vi "Create Message Classes for Actor.vi"(8 "error in (no error)":errorcluster, 11 "Object":T1) -> (0 "error out":errorcluster)   [LabVIEW 2020, in "Actor Message Maker Provider.lvlib"]
uses:
  Actor Message Maker Provider.lvlib
  MessageMakerProvider/Message Maker Provider.lvlib
  MessageMakerProvider/AFPP Shared/AFPP Shared.lvlib
  <vilib>/ErrorRing/Error Ring.xnode
  MessageMakerProvider/AFPP Shared/Validation Mode.ctl
  <vilib>/Utility/error.llb/Error Cluster From Error Code.vi
  <resource>/Framework/Providers/API/ItemRef.ctl
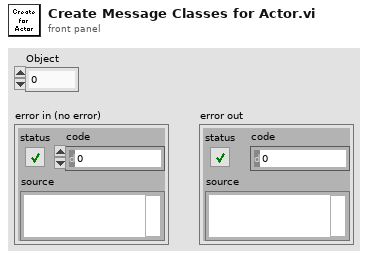
[diagram p1: front panel]
types:
  T1 = typedef "ItemRef.ctl" = u64
  T2 = typedef "AFPP Shared.lvlib/Validation Mode.ctl" = enum16{"An Actor Library", "A Target Tag"}
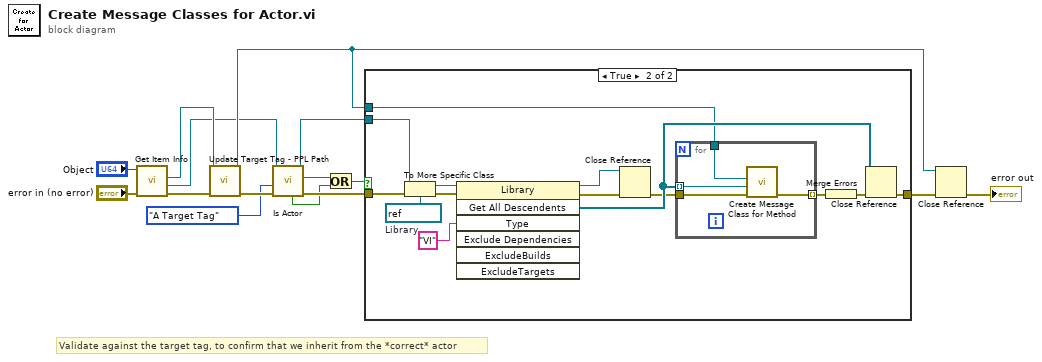
[diagram p0: block diagram]
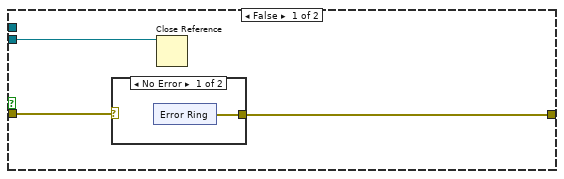
[diagram p2: hidden frame]
diagram:
  # "Validate against the target tag, to confirm that we inherit from the *correct* actor"
  n1 = call "Get Item Info.vi"("error in (no error)"="error in (no error)", "Object"="Object") -> ("error out"=w11:errorcluster, "Item Refnum"=w6:refnum<vi>, "Target"=w10:refnum<vi>)  [unwired: 5 in, 2 out]
  n2 = call "Update Target Tag - PPL Path.vi"("error in (no error)"=w11, "Target"=w10) -> ("error out"=w8:errorcluster, "dup Target"=w9:refnum<vi>)  [unwired: 7 in, 1 out]
  n3 = call "Is Actor.vi"("error in (no error)"=w8, "Validation"=Validation_Mode."A Target Tag", "ProjectItem in"=w6) -> ("error out"=w7:errorcluster, "Is Actor"=w2:bool, "ProjectItem out"=w5:refnum<vi>, "Is Actor Interface"=w1:bool)  [unwired: 4 in, 1 out]
  n4 = Or(x=w2, y=w1) -> (x .or. y?=w3:bool)
  n5 = case shown="True" w3 {
    tunnel: [w17 w33] -> w13
    tunnel: w9 -> [_ w28]
    tunnel: w7 -> [w18 w27]
    tunnel: w5 -> [w16 w26]
    frame False {
      n6 = case shown="No Error" w18 {
        selector: w18 -> [_ w25]
        tunnel: [w19 w25] -> w17
        frame No Error {
          n7 = xnode "Error Ring"() -> ("error out"=w19:errorcluster)
        }
        frame Error {
        }
      }
      n8 = Close Reference(reference=w16) -> ()  [unwired: 1 in, 1 out]
    }
    frame True {
      w39 = refnum<vi> refnum  # Library
      n9 = To More Specific Class(target class=w39, reference=w26, error in=w27) -> (specific class reference=w38:refnum<vi>, error out=w37:errorcluster)
      n10 = invoke class="Library" method="Get All Descendents"(reference=w38, error in=w37, "Type"="VI") -> (reference out=w35:refnum<vi>, error out=w30:errorcluster, "All Descendents"=w32:refnum<vi>[])  [unwired: 4 in, 4 out]
      n11 = Close Reference(reference=w35, error in (no error)=w30) -> (error out=w29:errorcluster)
      n12 = for {
        tunnel: w32 -> [w41] mode=indexing
        tunnel: w28 -> [w43]
        tunnel: w29 -> [w42]
        tunnel: [w40] -> w34 mode=indexing
        n13 = call "Create Message Class for Method.vi"("error in (no error)"=w42, "Item Refnum"=w41, "Target"=w43) -> ("error out"=w40:errorcluster)  [unwired: 6 in, 2 out]
      }
      n14 = Merge Errors(w34) -> (w31:errorcluster)
      n15 = Close Reference(reference=w32, error in (no error)=w31) -> (error out=w33:errorcluster)
    }
  }
  n16 = Close Reference(reference=w9, error in (no error)=w13) -> (error out=→"error out":errorcluster)
